vi "Continuous Measurement.vi"(8 "error in (no error)":errorcluster, 11 "Agilent 34401A in":refnum<class "Agilent 34401A.lvclass">) -> (0 "error out":errorcluster, 2 "Measured Value":dbl[](array[numeric]), 3 "Agilent 34401A out":refnum<class "Agilent 34401A.lvclass">)   [LabVIEW 2021, in "DMM.lvlib" / "Agilent 34401A.lvclass"]
uses:
  Agilent 34401A.lvclass
  C/Program Files (x86)/National Instruments/LabVIEW 2022/instr.lib/Agilent 34401/Public/Data/Read (Single Point).vi
panel:
  in  "Meas Setting":T1={"Function (0: DC Voltage)"=0, "Manual Resolution (5.5 Digits)"=5.5, "Manual Range (1.00)"=1.0, "Enable Auto Range (T: Enable)"=TRUE} {"Manual Range (1.00)" format="%_3f"; "Manual Resolution (5.5 Digits)" items=["4.5"=4.5, "5.5"=5.5, "6.5"=6.5]; "Function (0: DC Voltage)" items=["DC Voltage", "AC Voltage", "2 - Wire Resistance", "4 - Wire Resistance", "DC Current", "AC Current", "Frequency", "Period", "Continuity", "Diode Checking", "VDC:VDC Ratio", "Temperature", "Capacitance"]}
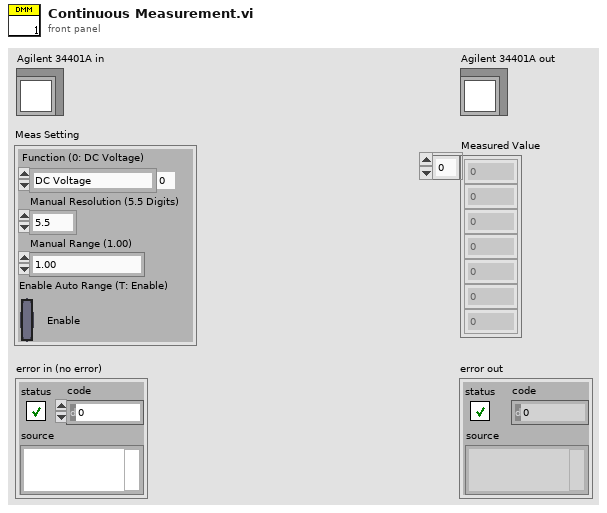
[diagram p1: front panel]
types:
  T1 = cluster{"Function (0: DC Voltage)":u16, "Manual Resolution (5.5 Digits)":dbl, "Manual Range (1.00)":dbl, "Enable Auto Range (T: Enable)":bool}
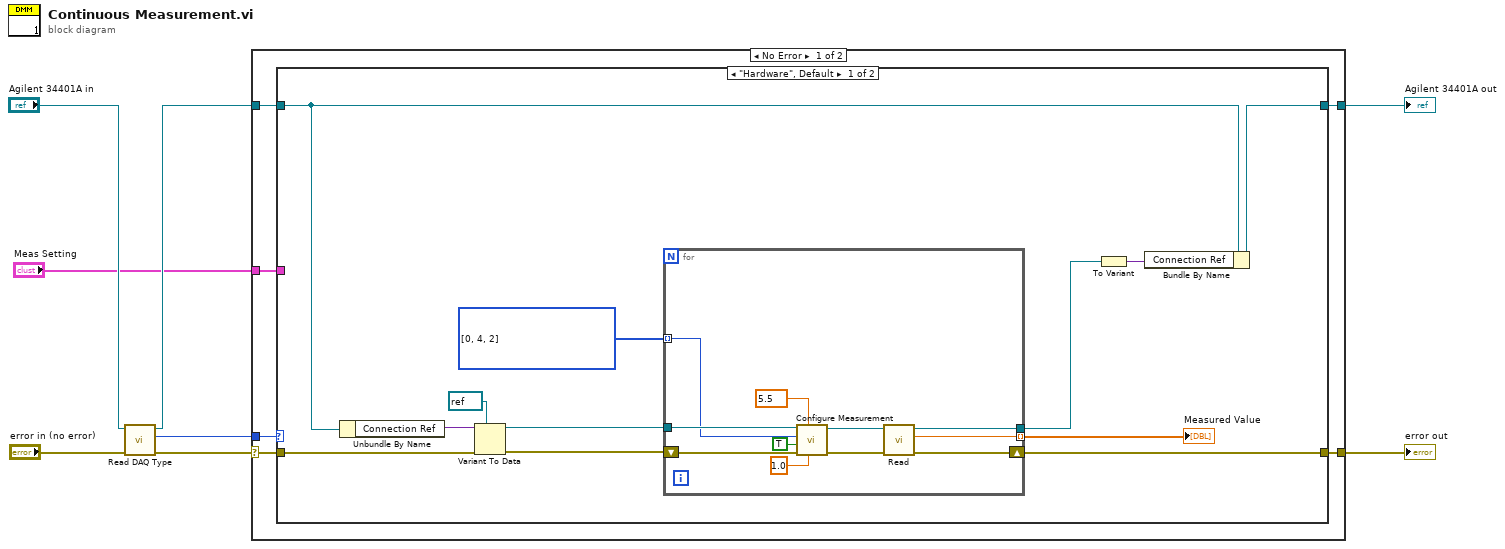
[diagram p0: block diagram]
diagram:
  n1 = call-dynamic "Read DAQ Type.vi"("error in (no error)"="error in (no error)", "Agilent 34401A in"="Agilent 34401A in") -> ("error out"=w5:errorcluster, "DAQ Type"=w2:enum16{"Hardware", "Simulation"}, "Agilent 34401A out"=w3:refnum<class "Agilent 34401A.lvclass">)  [unwired: 7 in]
  n2 = case shown="No Error" w5 {
    selector: w5 -> [w10 w40]
    tunnel: w3 -> [w13 w41]
    tunnel: [w12 w41] -> w7
    tunnel: [w9 w40] -> w6
    tunnel: w2 -> [w14 _]
    tunnel: "Meas Setting" -> [w11 _]
    frame No Error {
      n3 = case shown="\"Hardware\", Default" w14 {
        tunnel: w13 -> [w16 w39]
        tunnel: [w21 w39] -> w12
        tunnel: w11 -> [_ _]
        tunnel: w10 -> [w25 w38]
        tunnel: [w26 w38] -> w9
        frame "Hardware", Default {
          w22 = u16[] [0, 4, 2] items=["DC Voltage", "AC Voltage", "2 - Wire Resistance", "4 - Wire Resistance", "DC Current", "AC Current", "Frequency", "Period", "Continuity", "Diode Checking", "VDC:VDC Ratio", "Temperature", "Capacitance"]
          n4 = Unbundle By Name(w16) -> ("Connection Ref"=w15:variant)
          n5 = Variant To Data(error in=w25, type=refnum<visa-resource-name> refnum ("VISA resource name"), Variant=w15) -> (data=w23:refnum<visa-resource-name>, error out=w17:errorcluster)
          n6 = for {
            shift-right: [w35] -> w26
            shift-left: w17 -> [w37]
            tunnel: w23 -> [w34]
            tunnel: w22 -> [w33] mode=indexing
            tunnel: [w29] -> w18 mode=indexing
            tunnel: [w28] -> w20
            w32 = 5.5 items=["4.5"=4.5, "5.5"=5.5, "6.5"=6.5] ("Manual Resolution (5.5 Digits)")
            n7 = call "Configure Measurement.vi"("Manual Range (1.00)"=1.0, "Manual Resolution (5.5 Digits)"=w32, "error in (no error)"=w37, "Enable Auto Range (T: Enable)"=TRUE, "Function (0: DC Voltage)"=w33, "VISA resource name"=w34) -> ("error out"=w36:errorcluster, "VISA resource name out"=w30:refnum<visa-resource-name>)  [unwired: 4 in]
            n8 = call-poly "Read.vi"("error in (no error)"=w36, "VISA resource name"=w30) -> ("error out"=w35:errorcluster, "Measurement"=w29:dbl, "VISA resource name out"=w28:refnum<visa-resource-name>)  [unwired: 7 in]
          }
          "Measured Value" <- w18
          n9 = To Variant(anything=w20) -> (Variant=w19:variant)
          n10 = Bundle By Name(cluster=w16, "Connection Ref"=w19) -> (w21:refnum<class "Agilent 34401A.lvclass">)
        }
        frame "Simulation" {
        }
      }
    }
    frame Error {
    }
  }
  "error out" <- w6
  "Agilent 34401A out" <- w7
